vi "deploy directory.vi"(8 "error in (no error)":errorcluster, 10 "from path":path, 11 "to path":path) -> (0 "error out":errorcluster)   [LabVIEW 2014]
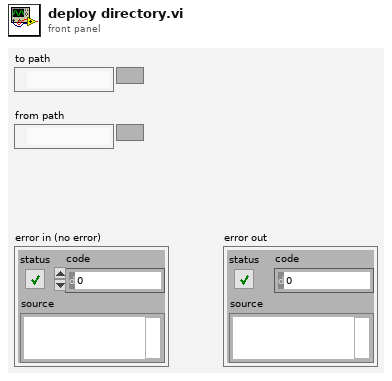
[diagram p1: front panel]
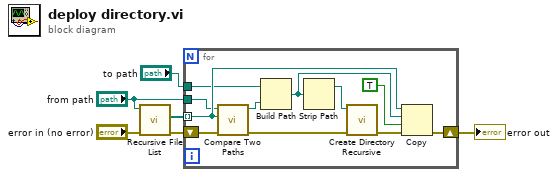
[diagram p0: block diagram]
diagram:
  n1 = call <vilib>:"Recursive File List.vi"("error in (no error)"="error in (no error)", "Folder Path"="from path") -> ("error out"=w3:errorcluster, "All Files in Dir"=w1:path[])  [unwired: 5 in, 3 out]
  n2 = for {
    tunnel: "to path" -> [w14]
    tunnel: w1 -> [w16] mode=indexing
    tunnel: "from path" -> [w15]
    shift-right: [w12] -> w6
    shift-left: w3 -> [w10]
    n3 = call <vilib>:"Compare Two Paths.vi"("error in (no error)"=w10, "Path 2"=w16, "Path 1"=w15) -> ("error out"=w9:errorcluster, "Relative Path from 1 to 2"=w13:path)  [unwired: 5 in, 2 out]
    n4 = Build Path(base path=w14, name or relative path=w13) -> (appended path=w11:path)
    n5 = Strip Path(path=w11) -> (stripped path=w8:path)  [unwired: 1 out]
    n6 = call <vilib>:"Create Directory Recursive.vi"("error in (no error)"=w9, "directory"=w8) -> ("error out"=w7:errorcluster)  [unwired: 3 in, 2 out]
    n7 = Copy(8:w7, 9:TRUE ("overwrite (F)"), 10:w11, 11:w16) -> (0:w12:errorcluster)  [unwired: 1 in, 2 out]
  }
  "error out" <- w6
